vi "Unify.vi"(6 "Core Actors":refnum<class "Actor.lvclass">[](array[class]), 9 "Mid Actors":refnum<class "Actor.lvclass">[](array[class]), 10 "Edge Actors":refnum<class "Actor.lvclass">[](array[class])) -> (1 "Unified Msgs":T1, 2 "Unified Actor":refnum<class "Actor.lvclass">)   [LabVIEW 2020, in "jettl.lvlib"]
uses:
  jettl.lvlib
  Actor/Actor.lvclass
  Msgs.ctl
  Msg/Msg.lvclass
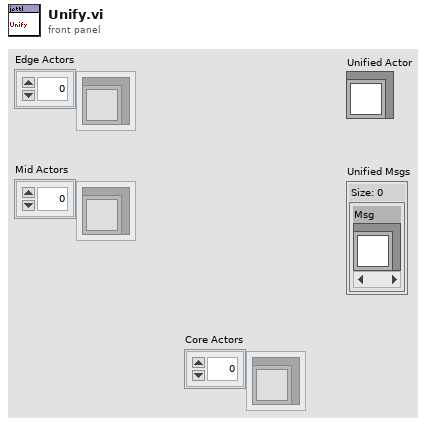
[diagram p1: front panel]
types:
  T1 = typedef "jettl.lvlib/Msgs.ctl" = set{refnum<class "Msg.lvclass">}
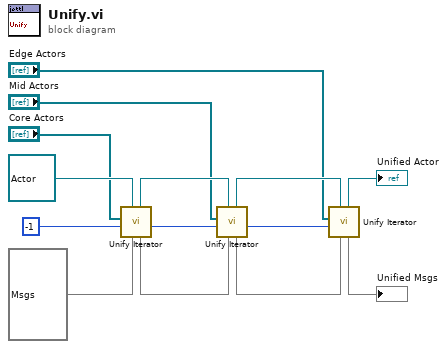
[diagram p0: block diagram]
diagram:
  n1 = call "Unify Iterator.vi"("Unified Msgs in"=T1 {}, "Actor in"=refnum<class "Actor.lvclass"> refnum, "Actor Index in"=-1, "Actors"="Core Actors") -> ("Actor Index out"=w5:i32, "Unified Msgs out"=w6:T1, "Actor out"=w11:refnum<class "Actor.lvclass">)  [unwired: 5 in]
  n2 = call "Unify Iterator.vi"("Unified Msgs in"=w6, "Actor in"=w11, "Actor Index in"=w5, "Actors"="Mid Actors") -> ("Actor Index out"=w4:i32, "Unified Msgs out"=w7:T1, "Actor out"=w10:refnum<class "Actor.lvclass">)  [unwired: 5 in]
  n3 = call "Unify Iterator.vi"("Unified Msgs in"=w7, "Actor in"=w10, "Actor Index in"=w4, "Actors"="Edge Actors") -> ("Unified Msgs out"=→"Unified Msgs":T1, "Actor out"=→"Unified Actor":refnum<class "Actor.lvclass">)  [unwired: 5 in, 1 out]
